vi "change byte order.vi"() -> ()   [LabVIEW 2019]
panel:
  out "Error Out":errorcluster
  in  "TDMS File":path=path "C:/Python/projects/nitdms/tests/tdms_files/change byte order.tdms"
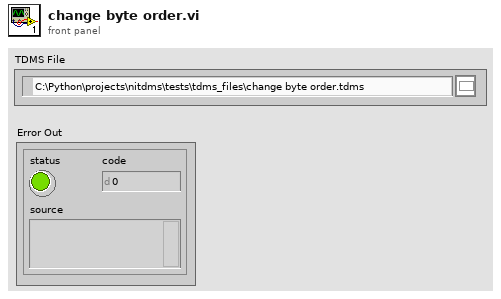
[diagram p1: front panel]
types:
  T1 = enum16{"big-endian, network order", "native, host order", "little-endian"}
  T2 = enum16{"open", "open or create", "create or replace", "create", "open (read-only)"}
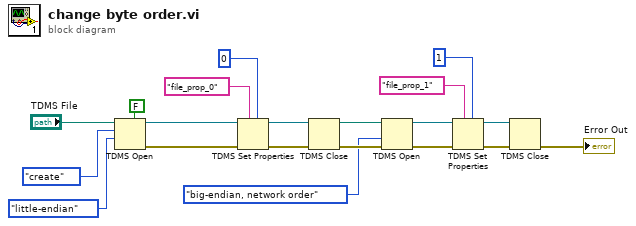
[diagram p0: block diagram]
diagram:
  n1 = TDMS Open(5:FALSE ("create index file? (T)"), 9:T1."little-endian" ("byte order (2:little-endian)"), 10:T2."create" ("operation (0:open)"), 11:"TDMS File") -> (0:w17:errorcluster, 3:w16:refnum<k34>)  [unwired: 3 in]
  n2 = TDMS Set Properties(5:0, 7:"file_prop_0", 8:w17, 11:w16) -> (0:w11:errorcluster, 3:w10:refnum<k34>)  [unwired: 2 in, 2 out]
  n3 = TDMS Close(8:w11, 11:w10) -> (0:w9:errorcluster, 3:w8:path)
  n4 = TDMS Open(8:w9, 9:T1."big-endian, network order" ("byte order (2:little-endian)"), 11:w8) -> (0:w5:errorcluster, 3:w4:refnum<k34>)  [unwired: 4 in]
  n5 = TDMS Set Properties(5:1, 7:"file_prop_1", 8:w5, 11:w4) -> (0:w3:errorcluster, 3:w2:refnum<k34>)  [unwired: 2 in, 2 out]
  n6 = TDMS Close(8:w3, 11:w2) -> (0:→"Error Out":errorcluster)  [unwired: 1 out]
